vi "Reentrant Method.vi"(8 "error in (no error)":errorcluster, 10 "Numeric":dbl, 11 "Test Interface Mock in":refnum<class "Test Interface Pure Mock.lvclass">) -> (0 "error out":errorcluster, 3 "Test Interface Mock out":refnum<class "Test Interface Pure Mock.lvclass">)   [LabVIEW 2020, in "Test Interface Pure Mock.lvclass"]
uses:
  Test Interface Pure Mock.lvclass
  C:/git/astemes-lmock/source/Framework/Pure Mock/Pure Mock.lvclass
  source/Framework/Pure Mock/Pure Mock.lvclass
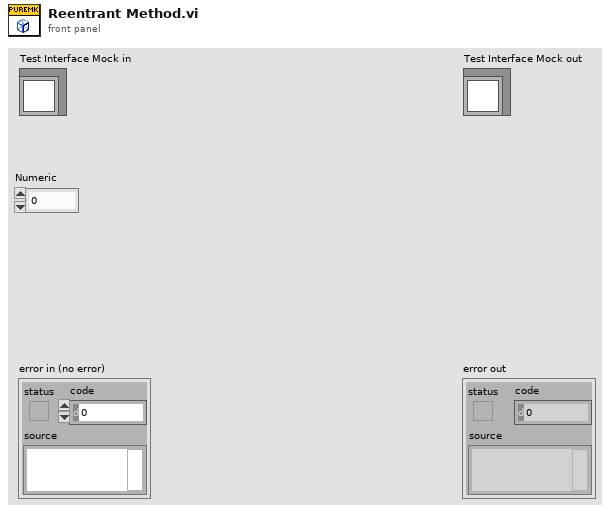
[diagram p1: front panel]
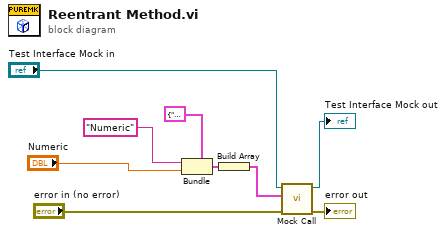
[diagram p0: block diagram]
diagram:
  n1 = Bundle(cluster=cluster{"Name":string, "Variant Data":variant} {"Name"="", "Variant Data"=variant}, "Name"="Numeric", "Variant Data"="Numeric") -> (w4:cluster{"Name":string, "Variant Data":variant})
  n2 = Build Array(w4) -> (w1:cluster{"Name":string, "Variant Data":variant}[])
  n3 = call "Mock Call.vi"("error in (no error)"="error in (no error)", "Control Values"=w1, "Mock In"="Test Interface Mock in") -> ("error out"=→"error out":errorcluster, "Mock Out"=→"Test Interface Mock out":refnum<class "Test Interface Pure Mock.lvclass">)  [unwired: 7 in]
